vi "Rec Destroy - Command.vi"(8 "error in (no error)":errorcluster, 11 "command-recordset reference":T1) -> (0 "error out":errorcluster, 3 "command reference":T2)   [LabVIEW 2017, in "NI_Database_API.lvlib"]
doc: "Frees an object by destroying its associated reference and returns a different reference object. Wire data to the reference input to determine the polymorphic instance to use or manually select the instance."
uses:
  <vilib>/addons/database/NI_Database_API.lvlib
  <vilib>/addons/database/Command.llb/Cmd ObjectReference.ctl
  <vilib>/addons/database/Command-Recordset.llb/Cmd-Rec Object Reference.ctl
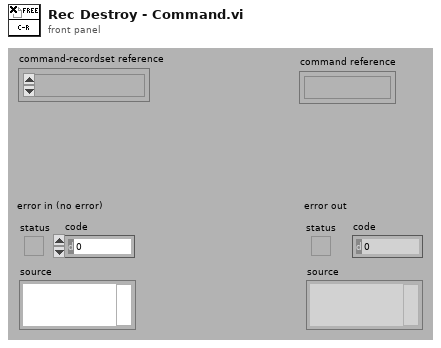
[diagram p1: front panel]
types:
  T1 = typedef "NI_Database_API.lvlib/Cmd-Rec Object Reference.ctl" = refnum<k1>
  T2 = typedef "NI_Database_API.lvlib/Cmd ObjectReference.ctl" = refnum<k1>
  T3 = typedef "NI_Database_API.lvlib/Rec ObjectReference.ctl" = refnum<k1>
  T4 = typedef "NI_Database_API.lvlib/Rec DataMembers.ctl" = cluster{"ADODB._Recordset":refnum<k7>, "Connection":T5}
  T5 = typedef "NI_Database_API.lvlib/Conn ObjectReference.ctl" = refnum<k1>
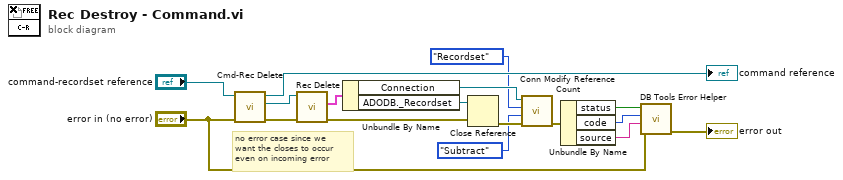
[diagram p0: block diagram]
diagram:
  # "no error case since we\nwant the closes to occur\neven on incoming error"
  n1 = call <vilib>:"Cmd-Rec Delete.vi"("error in (no error)"="error in (no error)", "command-recordset reference"="command-recordset reference") -> ("error out"=w6:errorcluster, "recordset reference"=w7:T3, "command reference"=→"command reference":T2)  [unwired: 3 out]
  n2 = call <vilib>:"Rec Delete.vi"("error in (no error)"=w6, "recordset reference"=w7) -> ("error out"=w12:errorcluster, "data"=w14:T4)  [unwired: 4 out]
  n3 = Unbundle By Name(w14) -> ("Connection"=w11:T5, "ADODB._Recordset"=w13:refnum<k7>)
  n4 = Close Reference(reference=w13, error in (no error)=w12) -> (error out=w10:errorcluster)
  n5 = call <vilib>:"Conn Modify Reference Count.vi"("error in (no error)"=w10, "operation"=enum16{"Add", "Subtract"}."Subtract" ("Operation"), "object"=enum16{"Recordset", "Command"}."Recordset" ("Object"), "connection reference"=w11) -> ("error out"=w2:errorcluster)  [unwired: 5 out]
  n6 = Unbundle By Name(w2) -> ("status"=w4:bool, "code"=w3:i32, "source"=w5:string)
  n7 = call <vilib>:"DB Tools Error Helper.vi"("Overriding error or warning"="error in (no error)", "source"=w5, "code"=w3, "status"=w4) -> ("error out"=→"error out":errorcluster)  [unwired: 7 out]
